vi "Begin.vi"() -> (3 "Номер образца 2":string="538")   [LabVIEW 2018]
panel:
  out "Boolean":bool=TRUE
  out "Ввел 2":bool=TRUE
  in  "Ввел":bool
  in  "Номер образца":string="0"
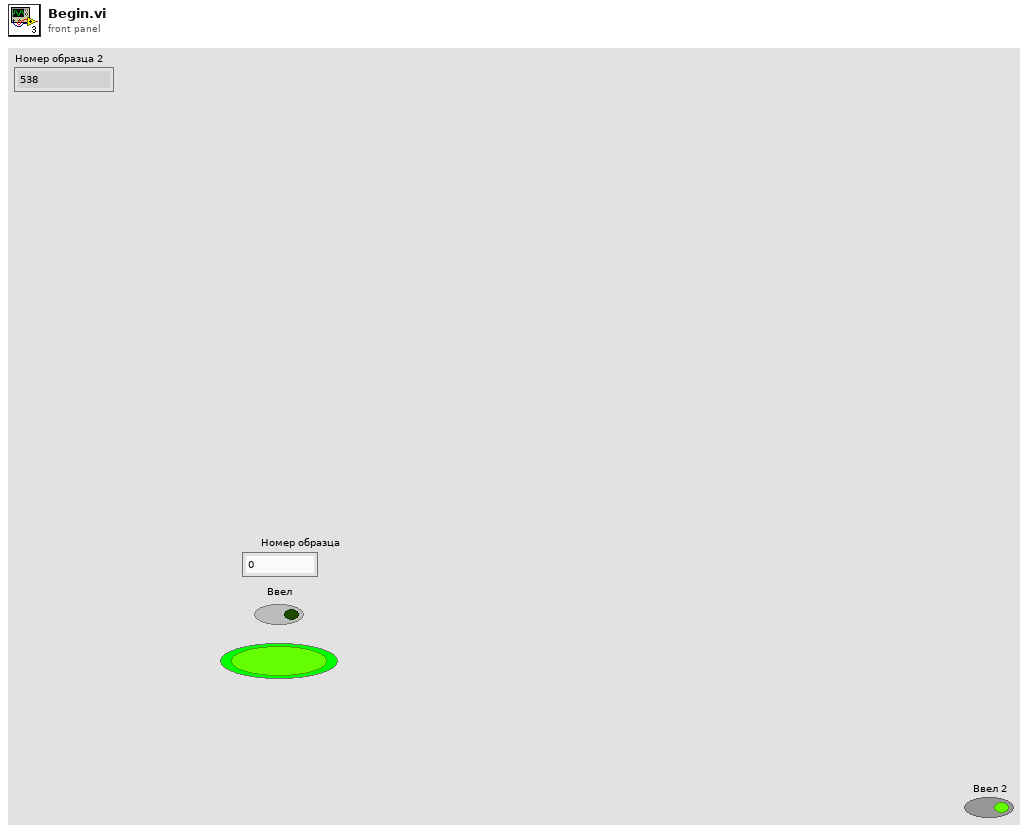
[diagram p1: front panel]
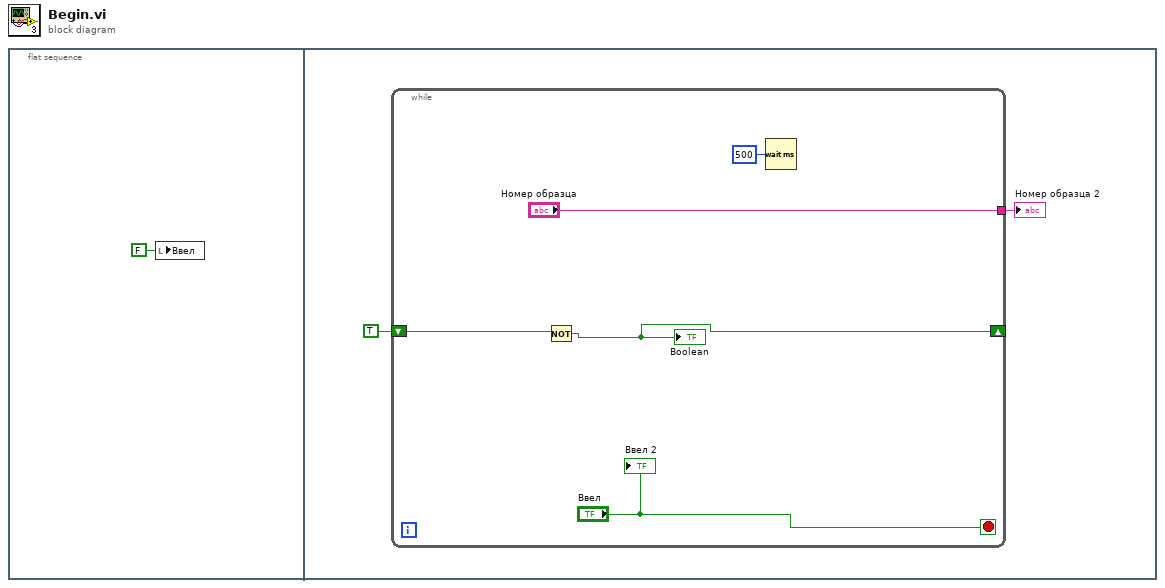
[diagram p0: block diagram]
diagram:
  n1 = flat-sequence {
    frame #0 {
      n2 = local write "Ввел"(FALSE ("Ввел")) -> ()
    }
    frame #1 {
      n3 = while {
        tunnel: ["Номер образца"] -> w3
        shift-right: [w4] -> _
        shift-left: TRUE -> [w5]
        stop <- "Ввел" stop-if-true
        n4 = Not(x=w5) -> (.not. x?=w4:bool)
        "Boolean" <- w4
        n5 = Wait (ms)(milliseconds to wait=u32 500) -> ()  [unwired: 1 out]
        "Ввел 2" <- "Ввел"
      }
      "Номер образца 2" <- w3
    }
  }
